vi "Write configuration.vi"(8 "error in":errorcluster, 10 "configuration":refnum<class "NISE_CEF_serializable configuration.lvclass">, 11 "NISE_CEF_serializable node folder in":refnum<class "NISE_CEF_serializable node folder.lvclass">) -> (0 "error out":errorcluster, 3 "NISE_CEF_serializable node folder out":refnum<class "NISE_CEF_serializable node folder.lvclass">)   [LabVIEW 2013, in "NISE_CEF_serializable node folder.lvclass"]
uses:
  NISE_CEF_serializable node folder.lvclass
  serializable configuration/NISE_CEF_serializable configuration.lvclass
  folder configuration/NISE_CEF_serializable node folder configuration.lvclass
  NISE_CEF_serializable node folder.lvclass/NISE_CEF_serializable node folder.ctl
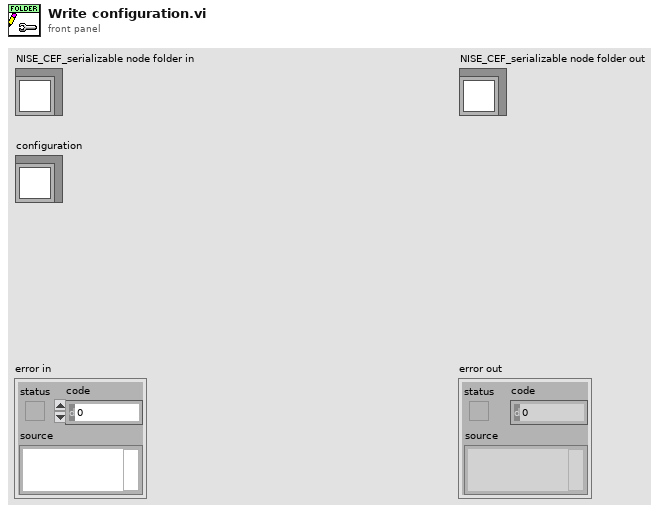
[diagram p1: front panel]
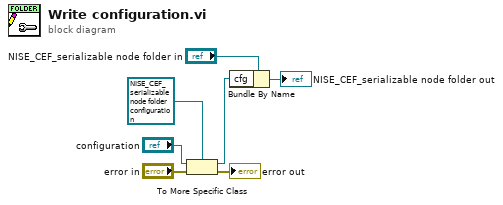
[diagram p0: block diagram]
diagram:
  n1 = To More Specific Class(target class=refnum<class "NISE_CEF_serializable node folder configuration.lvclass"> refnum ("folder configuration"), reference="configuration", error in="error in") -> (specific class reference=w1:refnum<class "NISE_CEF_serializable node folder configuration.lvclass">, error out=→"error out":errorcluster)
  n2 = Bundle By Name(cluster="NISE_CEF_serializable node folder in", "cfg"=w1) -> (→"NISE_CEF_serializable node folder out":refnum<class "NISE_CEF_serializable node folder.lvclass">)
